vi "DAQ Read Input.vi"(5 "error in":errorcluster, 6 "lines":tag) -> (1 "error out":errorcluster, 3 "task out":refnum<k21>)   [LabVIEW 2022 SP3]
uses:
  <vilib>/DAQmx/read.llb/DAQmx Read (Digital Bool 1Line 1Point).vi
  <vilib>/DAQmx/miscellaneous.llb/DAQmx Fill In Error Info.vi
panel:
  out "data":bool
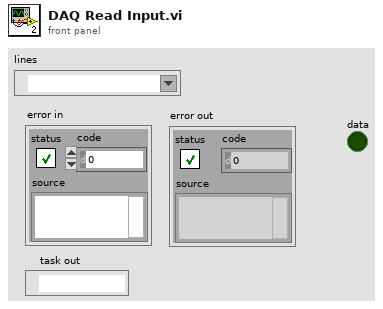
[diagram p1: front panel]
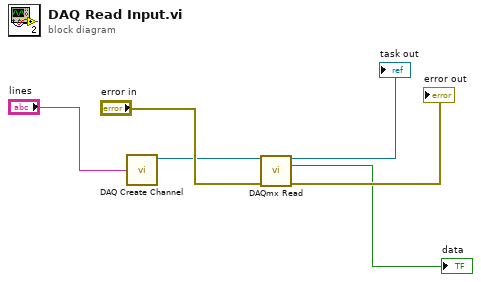
[diagram p0: block diagram]
diagram:
  n1 = call "DAQ Create Channel.vi"("lines"="lines") -> ("task out"=w3:refnum<k21>)  [unwired: 3 in, 1 out]
  n2 = call-poly <vilib>:"DAQmx Read.vi"("task/channels in"=w3, "error in"="error in") -> ("task out"=→"task out":refnum<k21>, "data"=→"data":bool, "error out"=→"error out":errorcluster)  [unwired: 11 in]
